vi "Frequency Control Master Table - Oversample.vi"() -> (1 "Sample Rate":dbl[](array[numeric]), 2 "Frequency":dbl[](array[numeric]), 3 "Table Index":dbl[](array[numeric]))   [LabVIEW 2010]
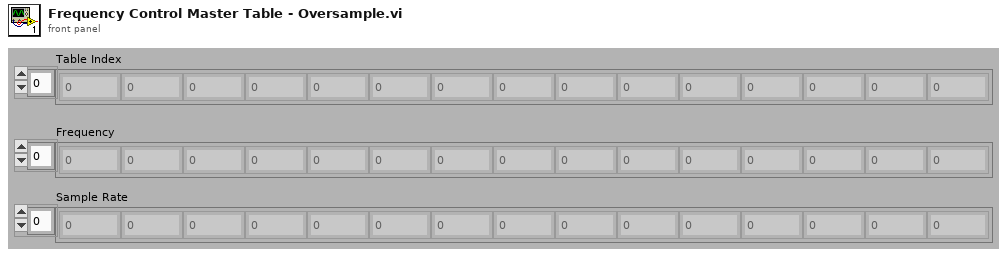
[diagram p1: front panel]
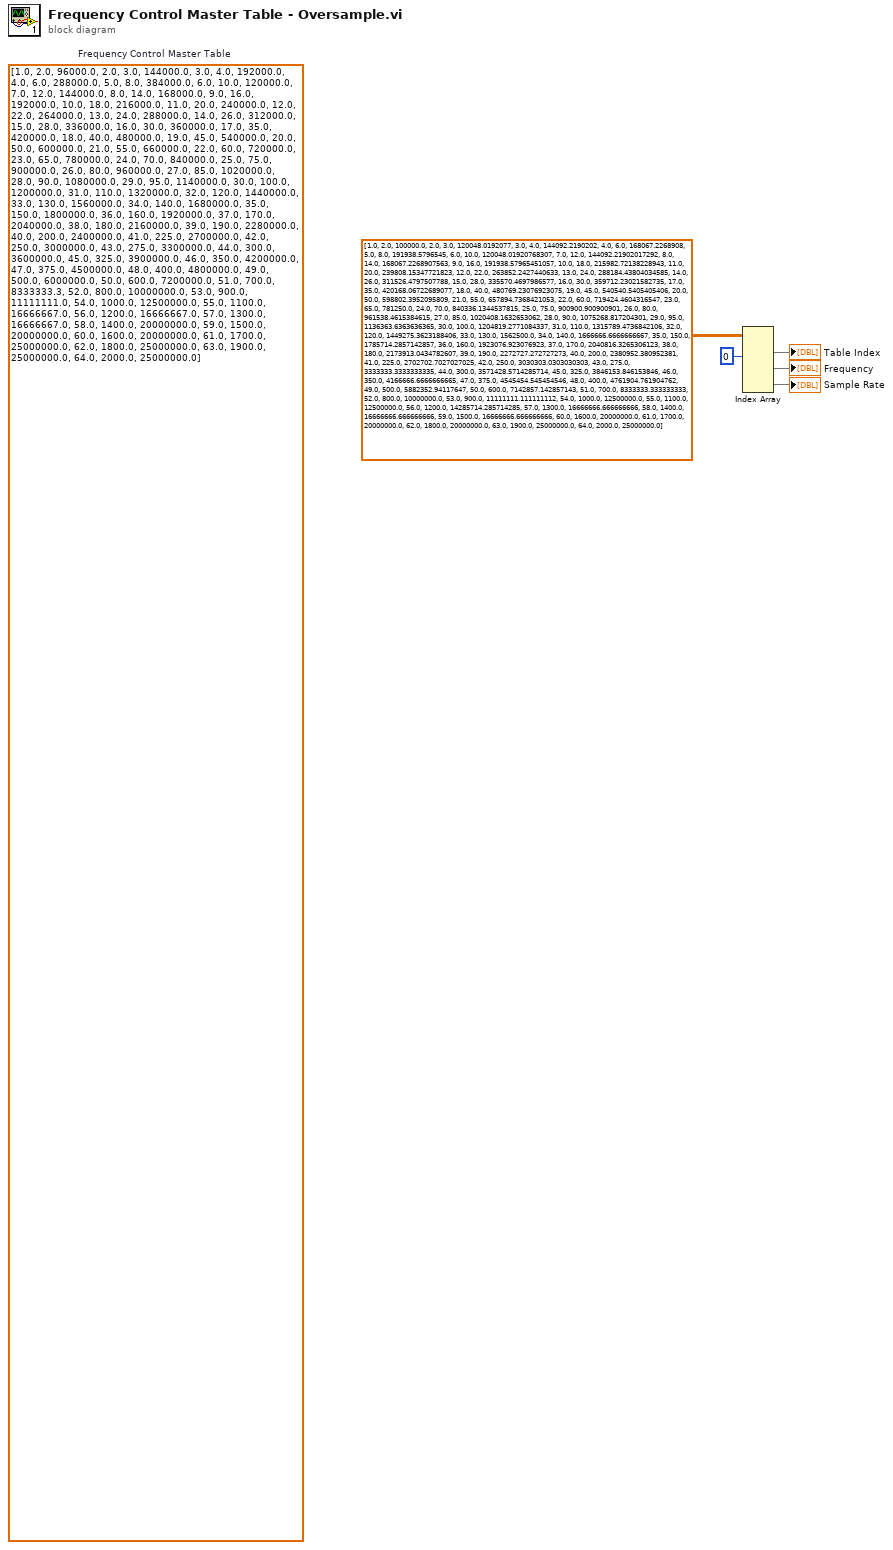
[diagram p0: block diagram]
diagram:
  (unwired) dbl[][] [[1.0, 2.0, 96000.0], [2.0, 3.0, 144000.0], [3.0, 4.0, 192000.0], [4.0, 6.0, 288000.0], [5.0, 8.0, 384000.0], [6.0, 10.0, 120000.0], [7.0, 12.0, 144000.0], [8.0, 14.0, 168000.0], [9.0, 16.0, 192000.0], [10.0, 18.0, 216000.0], [11.0, 20.0, 240000.0], [12.0, 22.0, 264000.0], [13.0, 24.0, 288000.0], [14.0, 26.0, 312000.0], [15.0, 28.0, 336000.0], [16.0, 30.0, 360000.0], [17.0, 35.0, 420000.0], [18.0, 40.0, 480000.0], [19.0, 45.0, 540000.0], [20.0, 50.0, 600000.0], [21.0, 55.0, 660000.0], [22.0, 60.0, 720000.0], [23.0, 65.0, 780000.0], [24.0, 70.0, 840000.0], [25.0, 75.0, 900000.0], [26.0, 80.0, 960000.0], [27.0, 85.0, 1020000.0], [28.0, 90.0, 1080000.0], [29.0, 95.0, 1140000.0], [30.0, 100.0, 1200000.0], [31.0, 110.0, 1320000.0], [32.0, 120.0, 1440000.0], [33.0, 130.0, 1560000.0], [34.0, 140.0, 1680000.0], [35.0, 150.0, 1800000.0], [36.0, 160.0, 1920000.0], [37.0, 170.0, 2040000.0], [38.0, 180.0, 2160000.0], [39.0, 190.0, 2280000.0], [40.0, 200.0, 2400000.0], [41.0, 225.0, 2700000.0], [42.0, 250.0, 3000000.0], [43.0, 275.0, 3300000.0], [44.0, 300.0, 3600000.0], [45.0, 325.0, 3900000.0], [46.0, 350.0, 4200000.0], [47.0, 375.0, 4500000.0], [48.0, 400.0, 4800000.0], [49.0, 500.0, 6000000.0], [50.0, 600.0, 7200000.0], [51.0, 700.0, 8333333.3], [52.0, 800.0, 10000000.0], [53.0, 900.0, 11111111.0], [54.0, 1000.0, 12500000.0], [55.0, 1100.0, 16666667.0], [56.0, 1200.0, 16666667.0], [57.0, 1300.0, 16666667.0], [58.0, 1400.0, 20000000.0], [59.0, 1500.0, 20000000.0], [60.0, 1600.0, 20000000.0], [61.0, 1700.0, 25000000.0], [62.0, 1800.0, 25000000.0], [63.0, 1900.0, 25000000.0], [64.0, 2000.0, 25000000.0]]  # Frequency Control Master Table
  n1 = Index Array(array=dbl[][] [[1.0, 2.0, 100000.0], [2.0, 3.0, 120048.0192077], [3.0, 4.0, 144092.2190202], [4.0, 6.0, 168067.2268908], [5.0, 8.0, 191938.5796545], [6.0, 10.0, 120048.01920768307], [7.0, 12.0, 144092.21902017292], [8.0, 14.0, 168067.2268907563], [9.0, 16.0, 191938.57965451057], [10.0, 18.0, 215982.72138228943], [11.0, 20.0, 239808.15347721823], [12.0, 22.0, 263852.2427440633], [13.0, 24.0, 288184.43804034585], [14.0, 26.0, 311526.4797507788], [15.0, 28.0, 335570.4697986577], [16.0, 30.0, 359712.23021582735], [17.0, 35.0, 420168.06722689077], [18.0, 40.0, 480769.23076923075], [19.0, 45.0, 540540.5405405406], [20.0, 50.0, 598802.3952095809], [21.0, 55.0, 657894.7368421053], [22.0, 60.0, 719424.4604316547], [23.0, 65.0, 781250.0], [24.0, 70.0, 840336.1344537815], [25.0, 75.0, 900900.900900901], [26.0, 80.0, 961538.4615384615], [27.0, 85.0, 1020408.1632653062], [28.0, 90.0, 1075268.817204301], [29.0, 95.0, 1136363.6363636365], [30.0, 100.0, 1204819.2771084337], [31.0, 110.0, 1315789.4736842106], [32.0, 120.0, 1449275.3623188406], [33.0, 130.0, 1562500.0], [34.0, 140.0, 1666666.6666666667], [35.0, 150.0, 1785714.2857142857], [36.0, 160.0, 1923076.923076923], [37.0, 170.0, 2040816.3265306123], [38.0, 180.0, 2173913.0434782607], [39.0, 190.0, 2272727.272727273], [40.0, 200.0, 2380952.380952381], [41.0, 225.0, 2702702.7027027025], [42.0, 250.0, 3030303.0303030303], [43.0, 275.0, 3333333.3333333335], [44.0, 300.0, 3571428.5714285714], [45.0, 325.0, 3846153.846153846], [46.0, 350.0, 4166666.6666666665], [47.0, 375.0, 4545454.545454546], [48.0, 400.0, 4761904.761904762], [49.0, 500.0, 5882352.94117647], [50.0, 600.0, 7142857.142857143], [51.0, 700.0, 8333333.333333333], [52.0, 800.0, 10000000.0], [53.0, 900.0, 11111111.111111112], [54.0, 1000.0, 12500000.0], [55.0, 1100.0, 12500000.0], [56.0, 1200.0, 14285714.285714285], [57.0, 1300.0, 16666666.666666666], [58.0, 1400.0, 16666666.666666666], [59.0, 1500.0, 16666666.666666666], [60.0, 1600.0, 20000000.0], [61.0, 1700.0, 20000000.0], [62.0, 1800.0, 20000000.0], [63.0, 1900.0, 25000000.0], [64.0, 2000.0, 25000000.0]] ("output array"), index (col) #1=0 ("disabled index (col)")) -> (element #1=→"Table Index":dbl[], element #2=→"Frequency":dbl[], element #3=→"Sample Rate":dbl[])  [unwired: 5 in]
